vi "GetAvailablePulseGenOutputLines.vi"(8 "error in (no error)":errorcluster, 11 "IMAQdx Session In":T1) -> (0 "error out":errorcluster, 2 "Available Output Lines":string[](array[string]), 3 "IMAQdx Session Out":T1)   [LabVIEW 2023]
uses:
  <vilib>/userdefined/High Color/IMAQdx.ctl
  <resource>/objmgr/imaqdx.rc
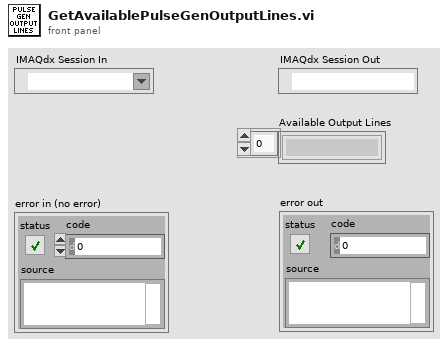
[diagram p1: front panel]
types:
  T1 = typedef "IMAQdx.ctl" = refnum<k21>
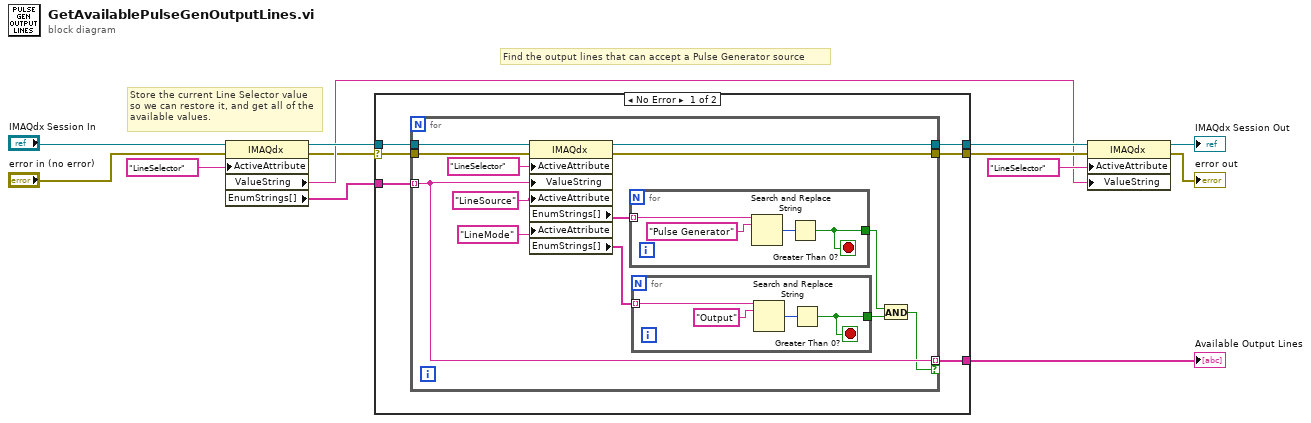
[diagram p0: block diagram]
diagram:
  # "Find the output lines that can accept a Pulse Generator source"
  # "Store the current Line Selector value so we can restore it, and get all of the available values."
  n1 = property class="IMAQdx"(reference="IMAQdx Session In", error in="error in (no error)", "ActiveAttribute"="LineSelector") -> (reference out=w12:T1, error out=w1:errorcluster, "ValueString"=w3:string, "EnumStrings[]"=w11:string[])
  n2 = case shown="No Error" w1 {
    selector: w1 -> [w14 w41]
    tunnel: w12 -> [w19 w42]
    tunnel: w11 -> [w18 _]
    tunnel: [w17 _] -> w10
    tunnel: [w16 w42] -> w6
    tunnel: [w15 w41] -> w4
    frame No Error {
      n3 = for {
        tunnel: w19 -> [w31]
        tunnel: w18 -> [w28] mode=indexing
        tunnel: [w28] -> w17 mode=indexing if=w20
        tunnel: [w27] -> w16
        tunnel: w14 -> [w26]
        tunnel: [w25] -> w15
        n4 = property class="IMAQdx"(reference=w31, error in=w26, "ActiveAttribute"="LineSelector", "ValueString"=w28, "ActiveAttribute"="LineSource", "ActiveAttribute"="LineMode") -> (reference out=w27:T1, error out=w25:errorcluster, "EnumStrings[]"=w29:string[], "EnumStrings[]"=w23:string[])
        n5 = for {
          tunnel: w29 -> [w40] mode=indexing
          tunnel: [w37] -> w21
          stop <- w37 stop-if-true
          n6 = Search and Replace String(input string=w40, search string="Pulse Generator") -> (number of replacements=w38:i32)  [unwired: 6 in, 3 out]
          n7 = Greater Than 0?(x=w38) -> (x > 0?=w37:bool)
        }
        n8 = for {
          tunnel: w23 -> [w36] mode=indexing
          tunnel: [w33] -> w22
          stop <- w33 stop-if-true
          n9 = Search and Replace String(input string=w36, search string="Output") -> (number of replacements=w34:i32)  [unwired: 6 in, 3 out]
          n10 = Greater Than 0?(x=w34) -> (x > 0?=w33:bool)
        }
        n11 = And(x=w21, y=w22) -> (x .and. y?=w20:bool)
      }
    }
    frame Error {
    }
  }
  "Available Output Lines" <- w10
  n12 = property class="IMAQdx"(reference=w6, error in=w4, "ActiveAttribute"="LineSelector", "ValueString"=w3) -> (reference out=→"IMAQdx Session Out":T1, error out=→"error out":errorcluster)
